vi "REV2mDistanceSensor Open.vi"(8 "MXP Profile":T1, 9 "Enable MXP (F)":bool, 10 "Onboard Profile":T1, 11 "Enable Onboard (F)":bool) -> (0 "error out":errorcluster, 3 "REV2mDistanceSensorsArray":T2={"Automatic Enabled"=TRUE, "Sensors[]"=[]})   [LabVIEW 2019, in "DistanceSensorDriver.lvlib"]
uses:
  DistanceSensorDriver.lvlib
  Typedef/Rev2mDistanceSensorsArray.ctl
  Typedef/REV2mDistanceSensorDevRef.ctl
  Typedef/Ports.ctl
  Typedef/RangeProfile.ctl
  Typedef/Ports_Inv.ctl
  Private/REV2mDistanceSensor Loop.vi
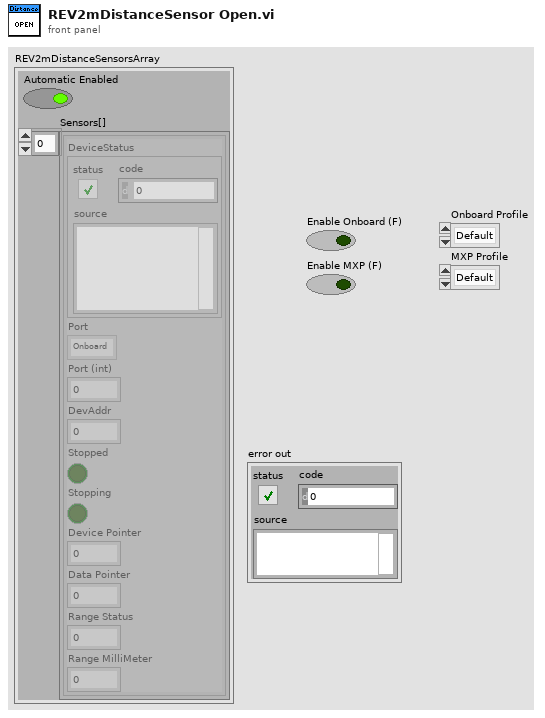
[diagram p1: front panel]
types:
  T1 = typedef "DistanceSensorDriver.lvlib/RangeProfile.ctl" = enum16{"Default", "High Speed", "High Accuracy", "Long Range"}
  T2 = typedef "DistanceSensorDriver.lvlib/Rev2mDistanceSensorsArray.ctl" = cluster{"Automatic Enabled":bool, "Sensors[]":T3[]}
  T3 = typedef "DistanceSensorDriver.lvlib/REV2mDistanceSensorDevRef.ctl" = cluster{"DeviceStatus":errorcluster, "Port":T4, "Port (int)":i32, "DevAddr":i32, "Stopped":bool, "Stopping":bool, "Device Pointer":u64, "Data Pointer":u64, "Range Status":u8, "Range MilliMeter":u16}
  T4 = typedef "DistanceSensorDriver.lvlib/Ports.ctl" = enum32{"Onboard", "MXP"}
  T5 = typedef "DistanceSensorDriver.lvlib/Ports_Inv.ctl" = enum16{"Onboard", "MXP", "Invalid"}
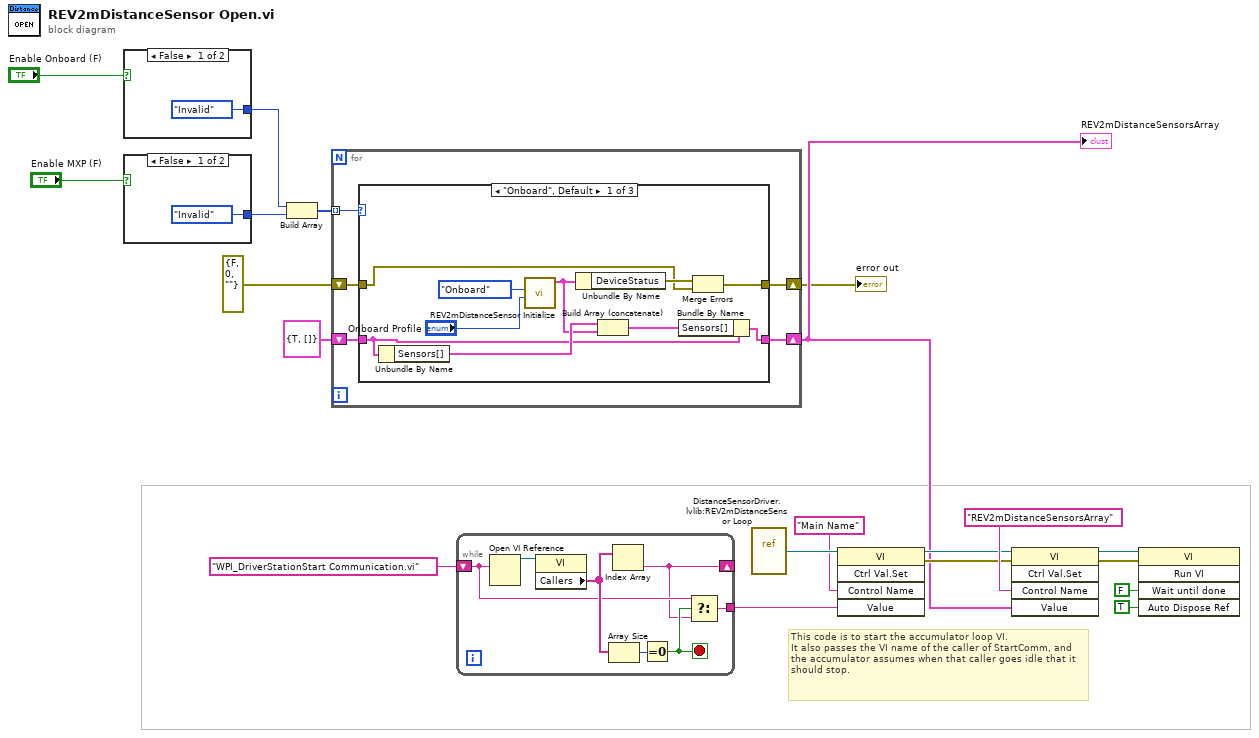
[diagram p0: block diagram]
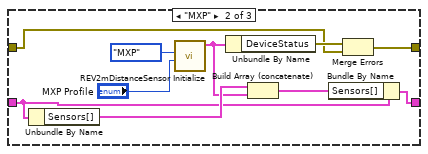
[diagram p2: hidden frame]
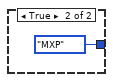
[diagram p4: hidden frame]
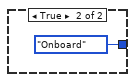
[diagram p5: hidden frame]
diagram:
  # "This code is to start the accumulator loop VI.\nIt also passes the VI name of the caller of StartComm, and the accumulator assumes when that caller goes idle that it should stop."
  n1 = case shown="False" "Enable Onboard (F)" {
    tunnel: [Ports_Inv."Invalid" ("Port_Inv") Ports_Inv."Onboard" ("Port_Inv")] -> w18
    frame False {
    }
    frame True {
    }
  }
  n2 = case shown="False" "Enable MXP (F)" {
    tunnel: [Ports_Inv."Invalid" ("Port_Inv") Ports_Inv."MXP" ("Port_Inv")] -> w17
    frame False {
    }
    frame True {
    }
  }
  n3 = Build Array(w18, w17) -> (w16:T5[])
  n4 = for {
    tunnel: w16 -> [w29] mode=indexing
    shift-right: [w28] -> w3
    shift-left: T2 {"Automatic Enabled"=TRUE, "Sensors[]"=[]} ("REV2mDistanceSensorsArray") -> [w27]
    shift-right: [w25] -> w1
    shift-left: errorcluster {"status"=FALSE, "code"=0, "source"=""} ("error constant") -> [w26]
    n5 = case shown="\"Onboard\", Default" w29 {
      tunnel: w27 -> [w37 w48 w51]
      tunnel: [w36 w46 w51] -> w28
      tunnel: w26 -> [w31 w41 w50]
      tunnel: [w30 w40 w50] -> w25
      frame "Onboard", Default {
        n6 = Unbundle By Name(w37) -> ("Sensors[]"=w38:T3[])
        n7 = call "REV2mDistanceSensor Initialize.vi"("Profile"="Onboard Profile", "Port"=Ports."Onboard") -> ("REV2mDistanceSensorDevRef Out"=w33:T3)  [unwired: 9 in]
        n8 = Unbundle By Name(w33) -> ("DeviceStatus"=w32:errorcluster)
        n9 = Build Array (concatenate)(w38, w33) -> (w39:T3[])
        n10 = Bundle By Name(cluster=w37, "Sensors[]"=w39) -> (w36:T2)
        n11 = Merge Errors(w32, w31) -> (w30:errorcluster)
      }
      frame "MXP" {
        n12 = Unbundle By Name(w48) -> ("Sensors[]"=w49:T3[])
        n13 = call "REV2mDistanceSensor Initialize.vi"("Profile"="MXP Profile", "Port"=Ports."MXP") -> ("REV2mDistanceSensorDevRef Out"=w42:T3)  [unwired: 9 in]
        n14 = Unbundle By Name(w42) -> ("DeviceStatus"=w43:errorcluster)
        n15 = Build Array (concatenate)(w49, w42) -> (w47:T3[])
        n16 = Bundle By Name(cluster=w48, "Sensors[]"=w47) -> (w46:T2)
        n17 = Merge Errors(w43, w41) -> (w40:errorcluster)
      }
      frame "Invalid" {
      }
    }
  }
  "REV2mDistanceSensorsArray" <- w3
  "error out" <- w1
  n18 = while {
    shift-right: [w53] -> _
    shift-left: "WPI_DriverStationStart Communication.vi" -> [w54]
    tunnel: [w52] -> w5
    stop <- w55 stop-if-true
    n19 = Open VI Reference(vi path=w54) -> (vi reference=w58:refnum<vi>)  [unwired: 1 in, 5 out]
    n20 = property class="VI"(reference=w58) -> ("Callers"=w56:string[])  [unwired: 1 in, 2 out]
    n21 = Array Size(array=w56) -> (size(s)=w57:i32)
    n22 = Index Array(array=w56) -> (element=w53:string)  [unwired: 1 in]
    n23 = Equal To 0?(x=w57) -> (x = 0?=w55:bool)
    n24 = Select(t=w54, s=w55, f=w53) -> (s? t:f=w52:string)
  }
  n25 = vi-ref "DistanceSensorDriver.lvlib:REV2mDistanceSensor Loop.vi"() -> (w7:refnum<vi>)
  n26 = invoke class="VI" method="Ctrl Val.Set"(reference=w7, "Control Name"="Main Name", "Value"=w5) -> (reference out=w4:refnum<vi>, error out=w9:errorcluster)  [unwired: 2 in, 3 out]
  n27 = invoke class="VI" method="Ctrl Val.Set"(reference=w4, error in=w9, "Control Name"="REV2mDistanceSensorsArray", "Value"=w3) -> (reference out=w14:refnum<vi>, error out=w10:errorcluster)  [unwired: 1 in, 3 out]
  n28 = invoke class="VI" method="Run VI"(reference=w14, error in=w10, "Wait until done"=FALSE ("Wait Until Done"), "Auto Dispose Ref"=TRUE ("Auto Dispose Reference")) -> ()  [unwired: 1 in, 5 out]
